vi "util_DoorInterface_cls_Unlock.vi"(0 "Interface_object in":refnum<class>, 5 "error in (no error)":errorcluster) -> (14 "Interface_object out":refnum<class>, 19 "error out":errorcluster)   [LabVIEW 2018, in "Timed Door.lvclass"]
uses:
  Timed Door.lvclass
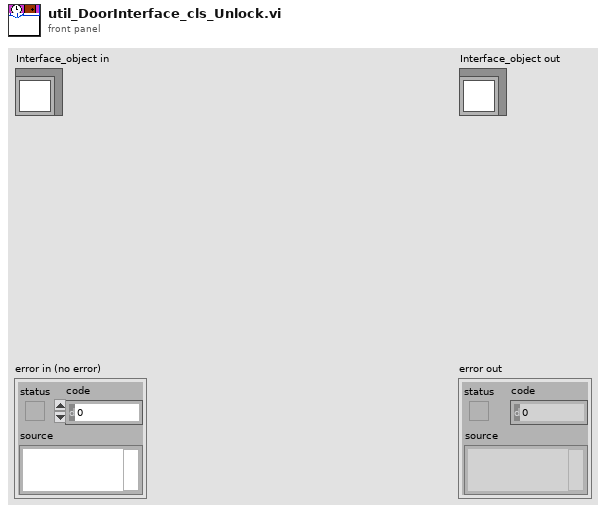
[diagram p1: front panel]
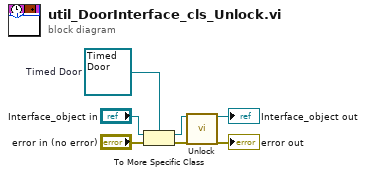
[diagram p0: block diagram]
diagram:
  w6 = refnum<class "Timed Door.lvclass"> refnum  # Timed Door
  n1 = To More Specific Class(target class=w6, reference="Interface_object in", error in="error in (no error)") -> (specific class reference=w4:refnum<class "Timed Door.lvclass">, error out=w5:errorcluster)
  n2 = call-dynamic "Unlock.vi"("Interface_object in"=w4, "error in (no error)"=w5) -> ("Interface_object out"=→"Interface_object out":refnum<class "Timed Door.lvclass">, "error out"=→"error out":errorcluster)  [unwired: 16 in]
